vi "Initialise.vi"(11 "Blink Period [s]":dbl) -> (3 "Blink out":refnum<class "Blinker.lvclass">)   [LabVIEW 2015, in "Blinker.lvclass"]
uses:
  Blinker.lvclass
  Blinker.lvclass/Blinker.ctl
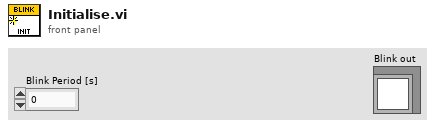
[diagram p1: front panel]
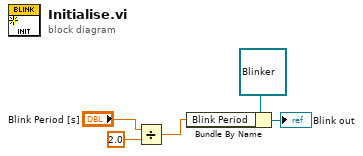
[diagram p0: block diagram]
diagram:
  n1 = Divide(x="Blink Period [s]", y=2.0) -> (x/y=w2:dbl)
  n2 = Bundle By Name(cluster=refnum<class "Blinker.lvclass"> refnum ("Blinker.lvclass"), "Blink Period"=w2) -> (→"Blink out":refnum<class "Blinker.lvclass">)
